vi "get_tack_points.vi"(7 "Obstacle Notifier":refnum<notifier>, 8 "NotifierReff":T1, 9 "Other leyline (deg)":dbl, 10 "Final leyline (deg)":dbl, 11 "Waypoint queue":refnum<queue>) -> (2 "Number of sailing points added":i32, 3 "Waypoint queue OUT":refnum<queue>)   [LabVIEW 2013]
uses:
  Data/TypeDefs/Notifiers.ctl
  Data/TypeDefs/UTM Location.ctl
  Data/TypeDefs/Sail Set Suggestions.ctl
  Data/TypeDefs/Rudder Set Suggestions.ctl
  Data/TypeDefs/OverrideInformation.ctl
  Data/TypeDefs/OverrideMode.ctl
  Data/TypeDefs/MotorSetup.ctl
  Data/TypeDefs/DynamixelSetupInfo.ctl
  Data/TypeDefs/AirmarStatus.ctl
  Data/TypeDefs/HardwareOnline.ctl
  Data/TypeDefs/DynamixelCycleTracker.ctl
  Data/TypeDefs/RC Input Values.ctl
  Classes/Waypoint/Waypoint.lvclass
  Classes/Obstacle/Obstacle.lvclass
  Utilities/Math/Angles/Angle/Angle.lvclass
panel:
  out "Proposed route will hit obstacles":bool
  out "Proposed WP array":refnum<class "Waypoint.lvclass">[](array[class])
  out "Number of full tack steps":i32
  out "Final tack step (m)":dbl
  in  "Amount to extend tack waypoints (m)":dbl=2.0
  # "TODO: Do something about this later"
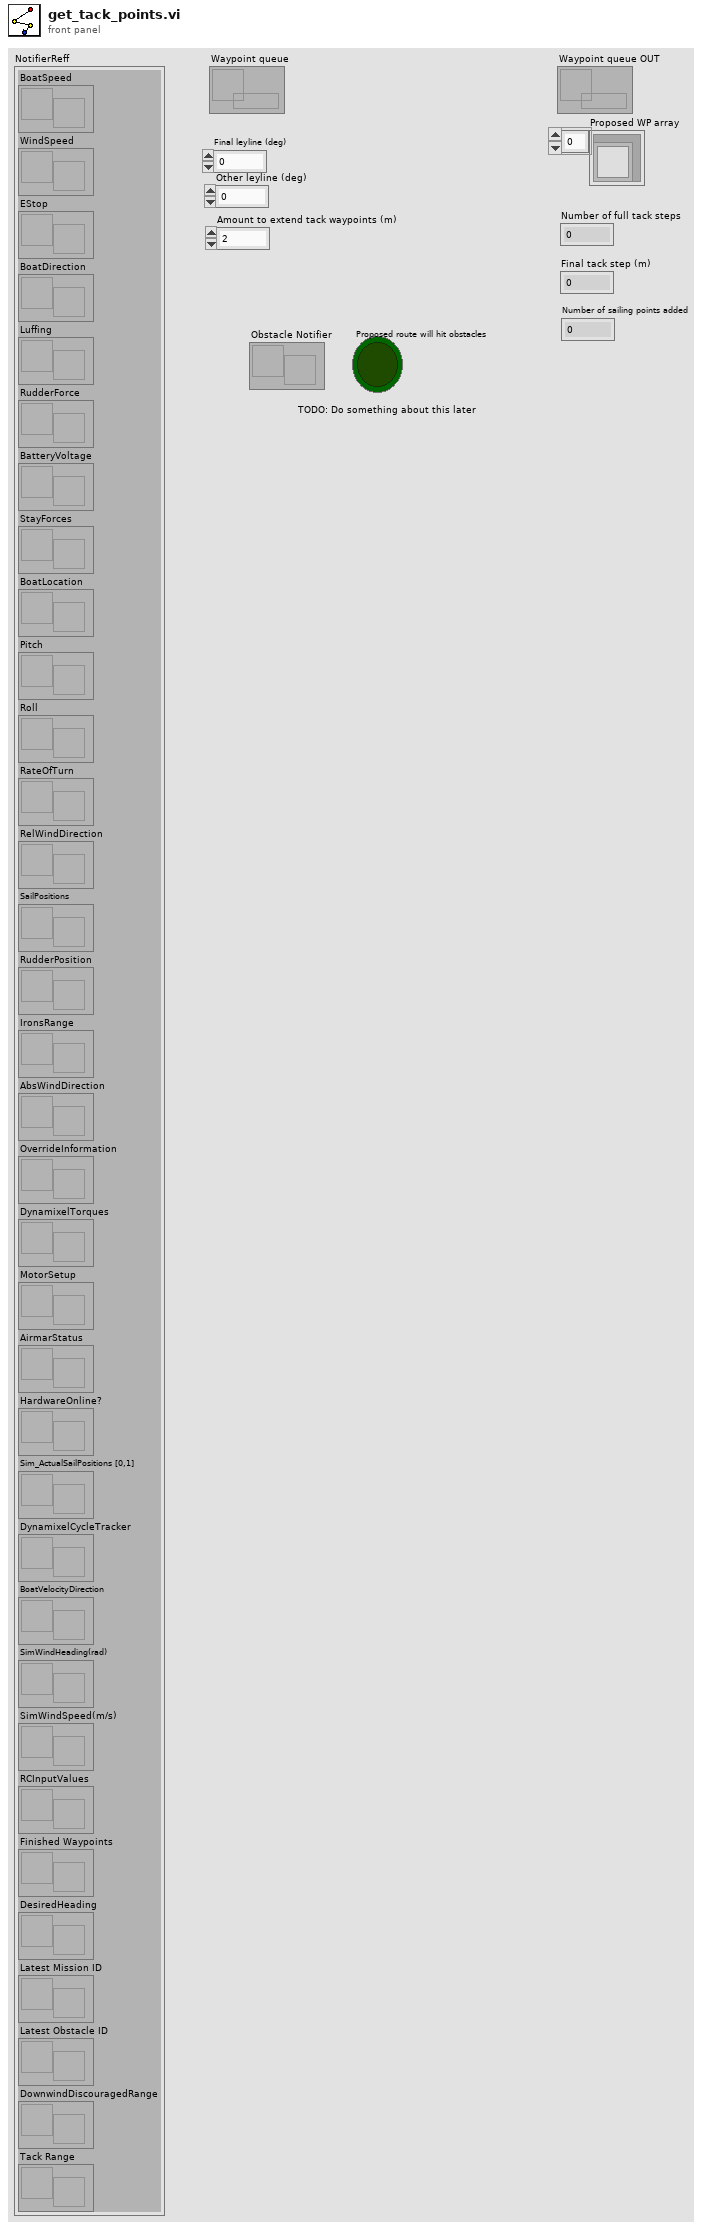
[diagram p1: front panel]
types:
  T1 = typedef "Notifiers.ctl" = cluster{"BoatSpeed":refnum<notifier>, "WindSpeed":refnum<notifier>, "EStop":refnum<notifier>, "BoatDirection":refnum<notifier>, "Luffing":refnum<notifier>, "RudderForce":refnum<notifier>, "BatteryVoltage":refnum<notifier>, "StayForces":refnum<notifier>, "BoatLocation":refnum<notifier>, "Pitch":refnum<notifier>, "Roll":refnum<notifier>, "RateOfTurn":refnum<notifier>, "RelWindDirection":refnum<notifier>, "SailPositions":refnum<notifier>, "RudderPosition":refnum<notifier>, "IronsRange":refnum<notifier>, "AbsWindDirection":refnum<notifier>, "OverrideInformation":refnum<notifier>, "DynamixelTorques":refnum<notifier>, "MotorSetup":refnum<notifier>, "AirmarStatus":refnum<notifier>, "HardwareOnline?":refnum<notifier>, "Sim_ActualSailPositions [0,1]":refnum<notifier>, "DynamixelCycleTracker":refnum<notifier>, "BoatVelocityDirection":refnum<notifier>, "SimWindHeading(rad)":refnum<notifier>, "SimWindSpeed(m/s)":refnum<notifier>, "RCInputValues":refnum<notifier>, "Finished Waypoints":refnum<notifier>, "DesiredHeading":refnum<notifier>, "Latest Mission ID":refnum<notifier>, "Latest Obstacle ID":refnum<notifier>, "DownwindDiscouragedRange":refnum<notifier>, "Tack Range":refnum<notifier>}
  T2 = typedef "UTM Location.ctl" = cluster{"UTM Zone":dbl, "Hemisphere":enum16{"North", "South"}, "East":dbl, "North":dbl}
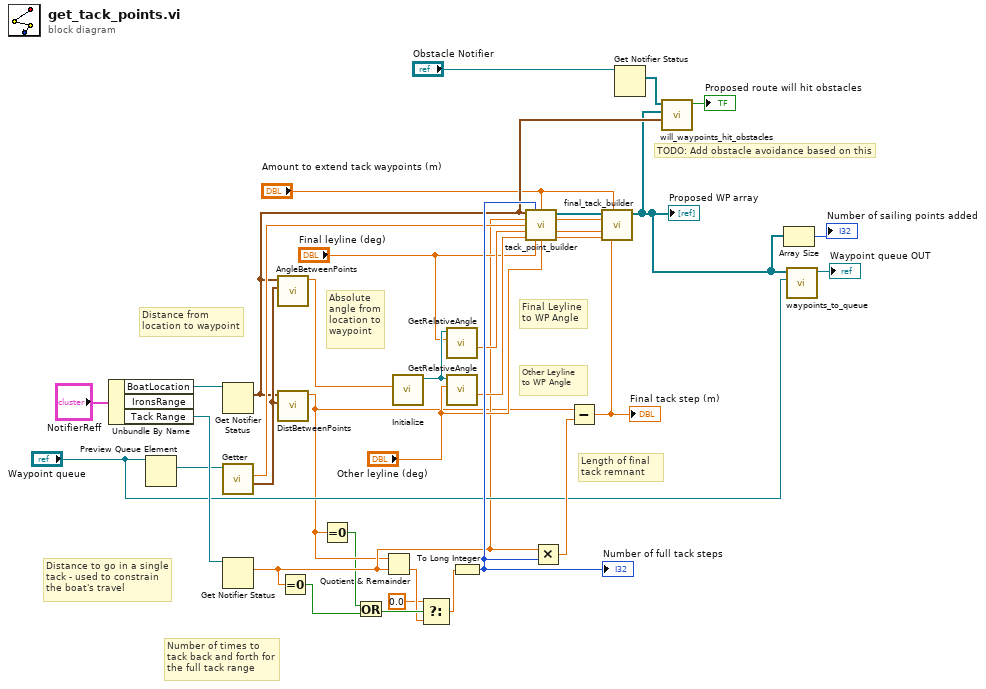
[diagram p0: block diagram]
diagram:
  # "TODO: Add obstacle avoidance based on this"
  # "Length of final tack remnant"
  # "Other Leyline to WP Angle"
  # "Final Leyline to WP Angle"
  # "Absolute angle from location to waypoint"
  # "Number of times to tack back and forth for the full tack range"
  # "Distance to go in a single tack - used to constrain the boat's travel"
  # "Distance from location to waypoint"
  n1 = Unbundle By Name("NotifierReff") -> ("BoatLocation"=w33:refnum<notifier>, "Tack Range"=w34:refnum<notifier>)  [unwired: 1 out]
  n2 = Preview Queue Element(queue="Waypoint queue") -> (element=w30:refnum<class "Waypoint.lvclass">)  [unwired: 2 in, 3 out]
  n3 = Get Notifier Status(notifier=w33) -> (current notification=w20:T2)  [unwired: 1 in, 4 out]
  n4 = call "Getter.vi"("Waypoint In"=w30) -> ("Coords"=w36:T2, "Tolerance (meters?)"=w27:dbl)  [unwired: 6 in, 3 out]
  n5 = Get Notifier Status(notifier=w34) -> (current notification=w8:dbl)  [unwired: 1 in, 4 out]
  n6 = call "AngleBetweenPoints.vi"("Point 2"=w36, "Point 1"=w20) -> ("Angle from P1 to P2"=w32:dbl)  [unwired: 9 in]
  n7 = call "DistBetweenPoints.vi"("UTM Location 2"=w36, "UTM Location 1"=w20) -> ("Distance from 1 to 2"=w7:dbl)  [unwired: 9 in]
  n8 = Equal To 0?(x=w8) -> (x = 0?=w5:bool)
  n9 = Equal To 0?(x=w7) -> (x = 0?=w6:bool)
  n10 = Or(x=w6, y=w5) -> (x .or. y?=w4:bool)
  n11 = Quotient & Remainder(x=w7, y=w8) -> (floor(x/y)=w3:dbl)  [unwired: 1 out]
  n12 = call "Initialize.vi"("Input Angle (Deg.)"=w32) -> ("Angle out"=w31:refnum<class "Angle.lvclass">)  [unwired: 9 in, 1 out]
  n13 = Select(t=0.0, s=w4, f=w3) -> (s? t:f=w2:dbl)
  n14 = call "GetRelativeAngle.vi"("Boat Heading (Deg.)"="Final leyline (deg)", "Angle in"=w31) -> ("Absolute difference (deg)"=w26:dbl)  [unwired: 6 in, 3 out]
  n15 = call "GetRelativeAngle.vi"("Boat Heading (Deg.)"="Other leyline (deg)", "Angle in"=w31) -> ("Absolute difference (deg)"=w25:dbl)  [unwired: 6 in, 3 out]
  n16 = To Long Integer(number=w2) -> (32bit integer=w28:i32)
  "Number of full tack steps" <- w28
  n17 = call "tack_point_builder.vi"("Boat Location"=w20, "Loop counts"=w28, "Amount to extend tack waypoints (m)"="Amount to extend tack waypoints (m)", "Distance for tack to travel (m)"=w8, "Tolerance (meters?)"=w27, "Angle (Final leyline -> WP) (deg)"=w26, "Angle (Other leyline -> WP) (deg)"=w25, "Final leyline (deg)"="Final leyline (deg)", "Other leyline (deg)"="Other leyline (deg)") -> ("Proposed WP array"=w19:refnum<class "Waypoint.lvclass">[], "Other leyline (deg)"=w18:dbl, "Angle (Final leyline -> WP) (deg) OUT"=w17:dbl, "Angle (Other leyline -> WP) (deg) OUT"=w16:dbl)  [unwired: 3 in]
  n18 = Multiply(x=w8, y=w28) -> (x*y=w29:dbl)
  n19 = Subtract(x=w7, y=w29) -> (x-y=w15:dbl)
  "Final tack step (m)" <- w15
  n20 = call "final_tack_builder.vi"("Distance for tack to travel (m)"=w15, "Amount to extend tack waypoints (m)"="Amount to extend tack waypoints (m)", "Angle (Other leyline -> WP) (deg)"=w16, "Angle (Final leyline -> WP) (deg)"=w17, "Other leyline (deg)"=w18, "Proposed WP array IN"=w19) -> ("Proposed WP array"=w10:refnum<class "Waypoint.lvclass">[])  [unwired: 5 in]
  "Proposed WP array" <- w10
  n21 = Get Notifier Status(notifier="Obstacle Notifier") -> (current notification=w21:refnum<class "Obstacle.lvclass">[])  [unwired: 1 in, 4 out]
  n22 = call "will_waypoints_hit_obstacles.vi"("Obstacle array"=w21, "WP array"=w10, "Boat Location"=w20) -> ("Will boat hit any obstacles?"=→"Proposed route will hit obstacles":bool)  [unwired: 7 in]
  n23 = Array Size(array=w10) -> (size(s)=→"Number of sailing points added":i32)
  n24 = call "waypoints_to_queue.vi"("Waypoint queue"="Waypoint queue", "WP array"=w10) -> ("Waypoint queue OUT"=→"Waypoint queue OUT":refnum<queue>)  [unwired: 9 in]
